vi "GetType.vi"(8 "error in (no error)":errorcluster, 11 "Configure Fixed Ref Junction [TC] Msg":refnum<class "Configure Fixed Ref Junction [TC] Msg.lvclass">) -> (0 "error out":errorcluster, 2 "Data Sample":variant, 3 "Configure Fixed Ref Junction [TC] Msg":refnum<class "Configure Fixed Ref Junction [TC] Msg.lvclass">)   [LabVIEW 2016, in "CS++DMM.lvlib" / "Configure Fixed Ref Junction [TC] Msg.lvclass"]
uses:
  Configure Fixed Ref Junction [TC] Msg.lvclass
  Configure Fixed Ref Junction [TC] Msg.lvclass/Configure Fixed Ref Junction [TC] Msg.ctl
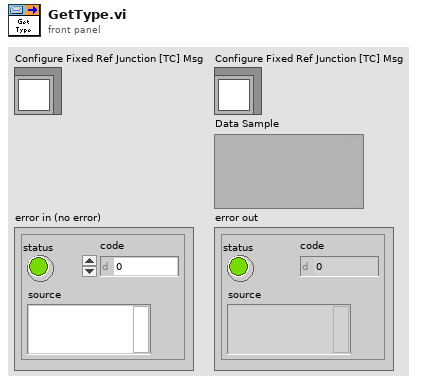
[diagram p1: front panel]
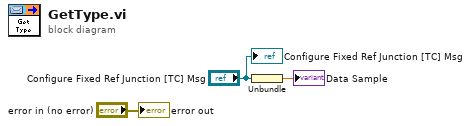
[diagram p0: block diagram]
diagram:
  n1 = Unbundle("Configure Fixed Ref Junction [TC] Msg") -> (→"Data Sample":dbl)
  "error out" <- "error in (no error)"
  "Configure Fixed Ref Junction [TC] Msg" <- "Configure Fixed Ref Junction [TC] Msg"
